vi "Intake.vi"(8 "error in (no error)":errorcluster, 9 "Out":bool, 10 "In":bool, 11 "Cargo in":refnum<class "Cargo.lvclass">) -> (0 "error out":errorcluster, 3 "Cargo out":refnum<class "Cargo.lvclass">)   [LabVIEW 2018, in "Cargo.lvlib" / "Cargo.lvclass"]
doc: "Use this VI to operate the intake"
uses:
  Cargo.lvclass
  Cargo.lvclass/Cargo.ctl
  Controls/Cargo States.ctl
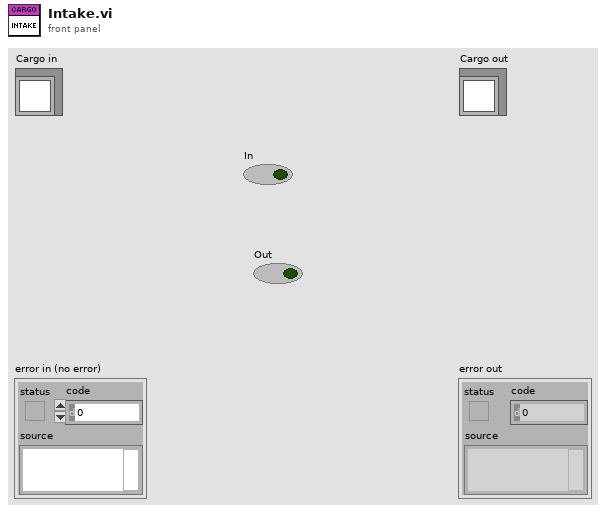
[diagram p1: front panel]
types:
  T1 = typedef "Cargo.lvlib/Cargo.lvclass/Cargo States.ctl" = enum16{"Off", "Intake Full", "Intake Idle", "Output Full"}
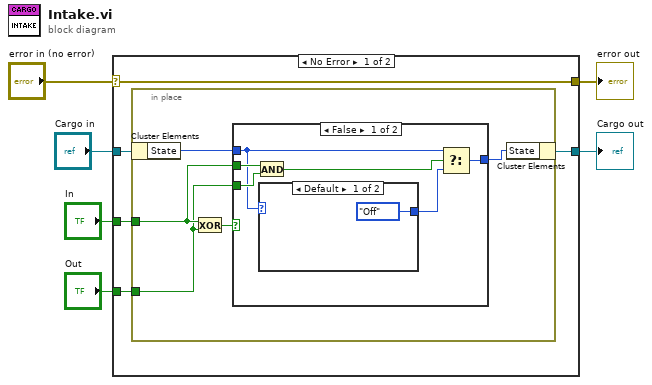
[diagram p0: block diagram]
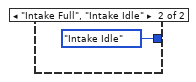
[diagram p2: hidden frame]
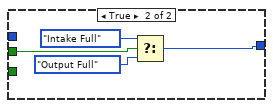
[diagram p3: hidden frame]
diagram:
  n1 = case shown="No Error" "error in (no error)" {
    selector: "error in (no error)" -> [w11 w30]
    tunnel: [w11 w30] -> w5
    tunnel: [w9 w29] -> w3
    tunnel: "Cargo in" -> [w10 w29]
    tunnel: "In" -> [w8 _]
    tunnel: "Out" -> [w7 _]
    frame No Error {
      n2 = in-place {
        in-place-border: w8 -> [w15]
        in-place-border: w7 -> [w13]
        n3 = in-place-cluster #1(w10) -> ("State"=w12:T1)
        n4 = Exclusive Or(1:w13, 2:w15) -> (0:w16:bool)
        n5 = case shown="False" w16 {
          tunnel: w15 -> [w22 w28]
          tunnel: [w19 w27] -> w14
          tunnel: w13 -> [w21 _]
          tunnel: w12 -> [w18 _]
          frame False {
            n6 = And(x=w22, y=w21) -> (x .and. y?=w20:bool)
            n7 = case shown="Default" w18 {
              tunnel: [Cargo_States."Off" ("State") Cargo_States."Intake Idle" ("State")] -> w17
              frame Default {
              }
              frame "Intake Full", "Intake Idle" {
              }
            }
            n8 = Select(t=w18, s=w20, f=w17) -> (s? t:f=w19:T1)
          }
          frame True {
            n9 = Select(t=Cargo_States."Intake Full" ("State"), s=w28, f=Cargo_States."Output Full" ("State")) -> (s? t:f=w27:T1)
          }
        }
        n10 = in-place-cluster #1("State"=w14) -> (w9:refnum<class "Cargo.lvclass">)
      }
    }
    frame Error {
    }
  }
  "error out" <- w5
  "Cargo out" <- w3
